vi "HEWH Mixing Valve ERD List.vi"(8 "error in (no error)":errorcluster, 11 "Disable Electronic Mixing Valve (EMV) List":bool) -> (0 "error out":errorcluster, 2 "Headers":string[](array[string]), 3 "Read ERD List":T1[](array[typedef]) {"ERD Number" format="%.0x"})   [LabVIEW 2016]
uses:
  type defs/ERD Read Data In.ctl
  type defs/Data Type.ctl
  library/GEA2_Toolkit.lvlib
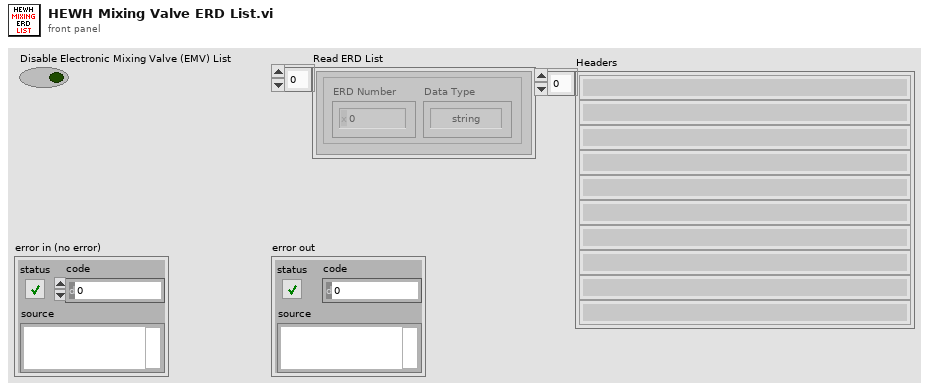
[diagram p1: front panel]
types:
  T1 = typedef "GEA2_Toolkit.lvlib/ERD Read Data In.ctl" = cluster{"ERD Number":u16, "Data Type":T2}
  T2 = typedef "GEA2_Toolkit.lvlib/Data Type.ctl" = enum16{"string", "boolean", "uint8_t", "uint16_t", "uint32_t", "uint64_t"}
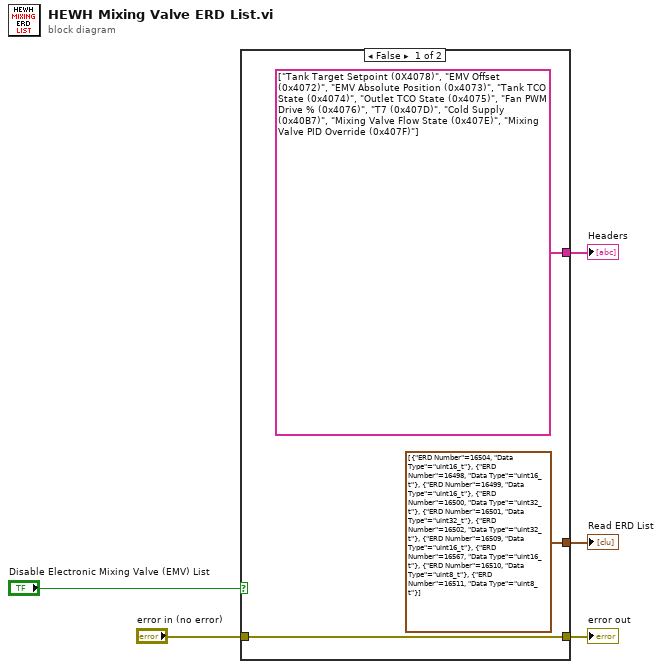
[diagram p0: block diagram]
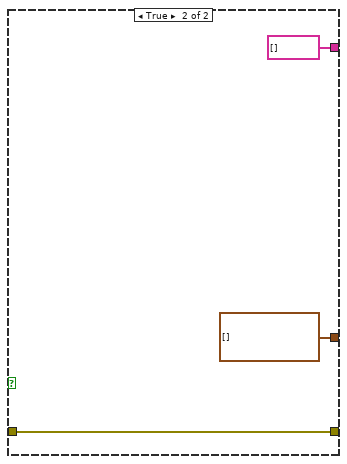
[diagram p2: hidden frame]
diagram:
  n1 = case shown="False" "Disable Electronic Mixing Valve (EMV) List" {
    tunnel: [T1[] [{"ERD Number"=16504, "Data Type"=enum."uint16_t"}, {"ERD Number"=16498, "Data Type"=enum."uint16_t"}, {"ERD Number"=16499, "Data Type"=enum."uint16_t"}, {"ERD Number"=16500, "Data Type"=enum."uint32_t"}, {"ERD Number"=16501, "Data Type"=enum."uint32_t"}, {"ERD Number"=16502, "Data Type"=enum."uint32_t"}, {"ERD Number"=16509, "Data Type"=enum."uint16_t"}, {"ERD Number"=16567, "Data Type"=enum."uint16_t"}, {"ERD Number"=16510, "Data Type"=enum."uint8_t"}, {"ERD Number"=16511, "Data Type"=enum."uint8_t"}] ("Read ERD List") T1[] [] ("Read ERD List")] -> w5
    tunnel: "error in (no error)" -> [w7 w11]
    tunnel: [w7 w11] -> w2
    tunnel: [string[] ["Tank Target Setpoint (0X4078)", "EMV Offset (0x4072)", "EMV Absolute Position (0x4073)", "Tank TCO State (0x4074)", "Outlet TCO State (0x4075)", "Fan PWM Drive % (0x4076)", "T7 (0x407D)", "Cold Supply (0x40B7)", "Mixing Valve Flow State (0x407E)", "Mixing Valve PID Override (0x407F)"] string[] [] ("array")] -> w4
    frame False {
    }
    frame True {
    }
  }
  "Read ERD List" <- w5
  "Headers" <- w4
  "error out" <- w2
